vi "ARRAY1DHandle.vi"() -> ()   [LabVIEW 2023]
doc: "This function gets the floor of the square of all element values in input and returns them in output. This VI demonstrates preallocating array memory for a separate, returned array.\n\nFor information on the data types used for the DLL function, right-click on the Call Library Function node and choose Configure."
uses:
  CLF_Example.dll
panel:
  out "output":i32[](array[numeric])
  in  "input":dbl[](array[numeric])=[1.11, 2.22, 3.33, 4.44]
  # "See the block diagram for more information."
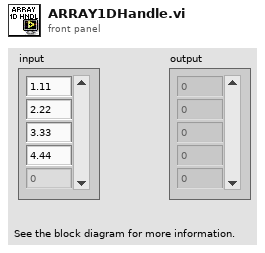
[diagram p1: front panel]
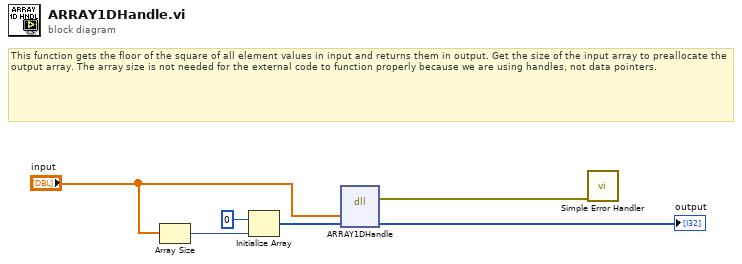
[diagram p0: block diagram]
diagram:
  # "This function gets the floor of the square of all element values in input and returns them in output. Get the size of the input array to preallocate the output array. The array size is not needed for the external code to function properly because we are using handles, not data pointers."
  n1 = Array Size(array="input") -> (size(s)=w4:i32)
  n2 = Initialize Array(0, w4) -> (w3:i32[])
  n3 = dll-call lib="c:/dev/_r/4/eng/lv-core/lvpostprocessingd/lv_mc_x86_64/dist_i386/examples/Connectivity/Libraries and Executables/DLL Calling VIs/CLF_Example**.*" fn="ARRAY1DHandle"("input"="input", "output"=w3) -> (error out=w1:errorcluster, "output"=→"output":i32[])  [unwired: 4 in, 2 out]
  n4 = call <vilib>:"Simple Error Handler.vi"("error in (no error)"=w1) -> ()  [unwired: 4 in, 5 out]
